vi "Host_SinglePointSuspension.vi"() -> ()   [LabVIEW 2024]
uses:
  <vilib>/FPGAPlugInAG/USB-7845R OEM/niLvFpga_Open_USB-7845R OEM.vi
  <vilib>/rvi/interface/common/dynamic/niFpgaDynamicAddResources.vi
  <vilib>/Utility/error.llb/Error Cluster From Error Code.vi
  <vilib>/rvi/errors/niLvFpgaAdjustHostInterfaceError.vi
  <vilib>/FPGAPlugInAG/Dynamic/niLvFpga_Close_Dynamic.vi
  <vilib>/rvi/interface/nirviOpenFPGA/nirviOpenFPGA.xnode
  FPGA Bitfiles/hoppingsicmv2_FPGATarget_FPGASinglePointS_HFntAzq5sS4.lvbitx
  <vilib>/rvi/interface/nirviReadWriteControl/nirviReadWriteControl.xnode
  <vilib>/rvi/interface/nirviCloseFPGA/nirviCloseFPGA.xnode
  NiFpgaLv.dll
  <vilib>/rvi/interface/Simulation/niFpgaSimulationCallBeginRW.vi
panel:
  in  "stop":bool
  in  "RetRate um/s":dbl format="%#_13g"
  in  "AppRate um/s":dbl format="%#_13g"
  in  "Retract um":dbl format="%#_13g"
  in  "Threshold %":dbl format="%#_13g"
  in  "Y um":dbl format="%#_13g"
  in  "X um":dbl format="%#_13g"
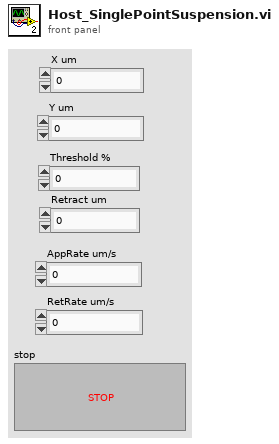
[diagram p1: front panel]
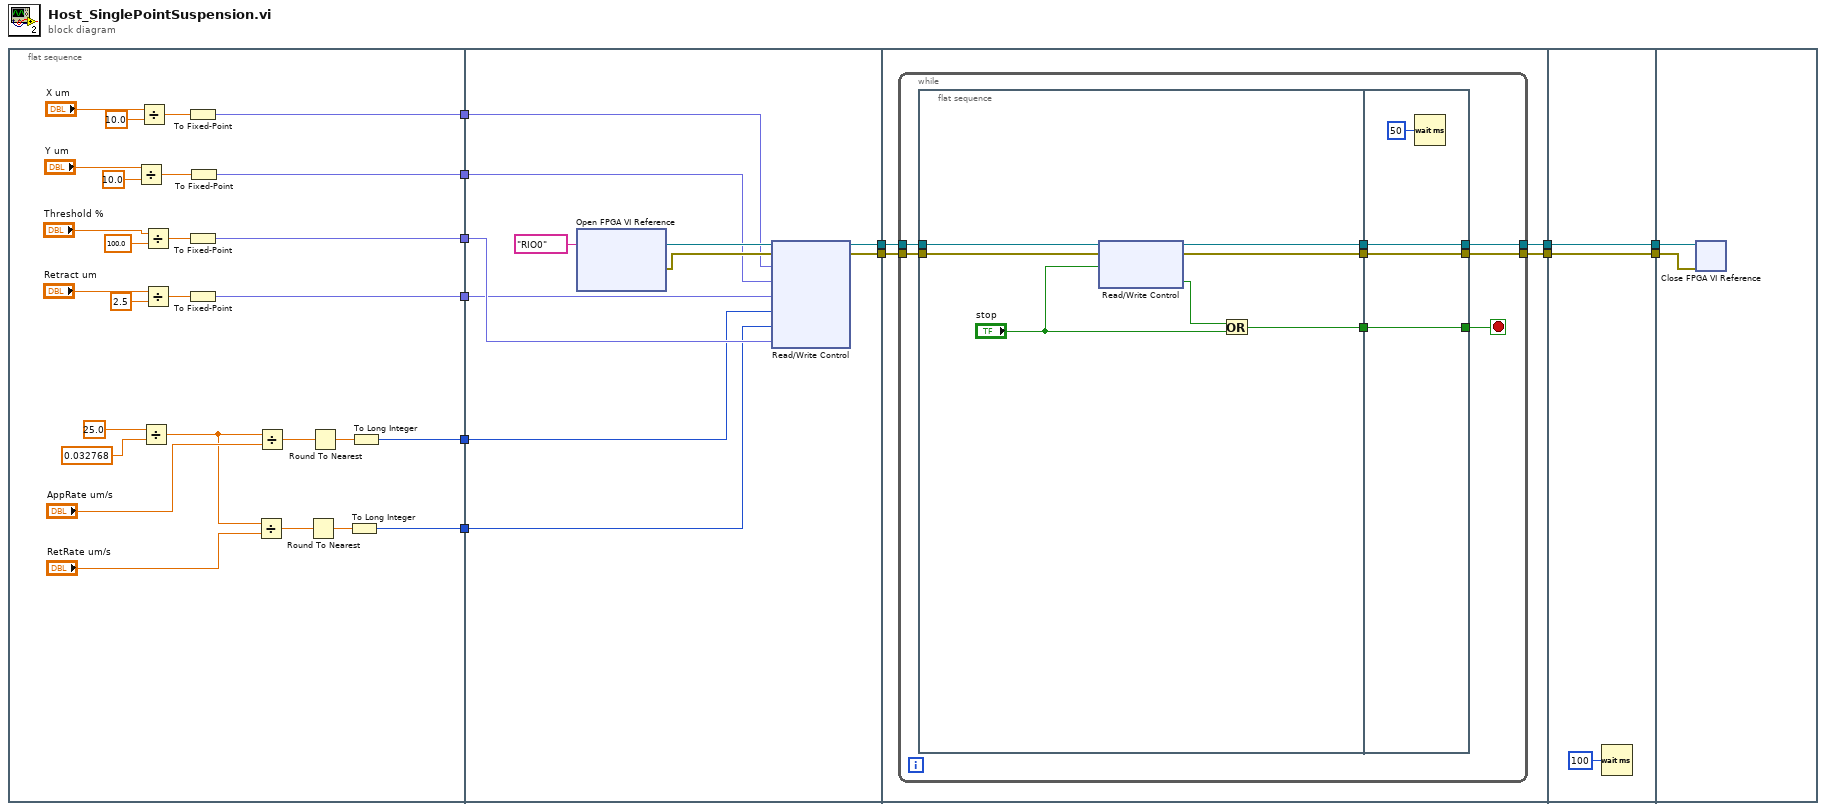
[diagram p0: block diagram]
diagram:
  n1 = flat-sequence {
    tunnel: [w36] -> w12
    tunnel: [w29] -> w11
    tunnel: [w28] -> w10
    tunnel: [w24] -> w9
    tunnel: [w14] -> w8
    tunnel: [w13] -> w7
    tunnel: w12 -> [w47]
    tunnel: w11 -> [w46]
    tunnel: w10 -> [w45]
    tunnel: w9 -> [w44]
    tunnel: w8 -> [w43]
    tunnel: w7 -> [w42]
    tunnel: [w41] -> w6
    tunnel: [w40] -> w5
    tunnel: w6 -> [w54]
    tunnel: w5 -> [w53]
    tunnel: [w52] -> w4
    tunnel: [w51] -> w3
    tunnel: w4 -> [w75]
    tunnel: w3 -> [w74]
    tunnel: [w75] -> w2
    tunnel: [w74] -> w1
    tunnel: w2 -> [w78]
    tunnel: w1 -> [w77]
    frame #0 {
      n2 = Divide(x="Y um", y=10.0) -> (x/y=w31:dbl)
      n3 = Divide(x="X um", y=10.0) -> (x/y=w30:dbl)
      n4 = Divide(x=25.0, y=0.032768) -> (x/y=w20:dbl)
      n5 = Divide(x="Threshold %", y=100.0) -> (x/y=w37:dbl)
      n6 = Divide(x="Retract um", y=2.5) -> (x/y=w27:dbl)
      n7 = To Fixed-Point(number=w30) -> (fixed-point=w29:fxp<+/-,48,16>)  [unwired: 1 in]
      n8 = To Fixed-Point(number=w37) -> (fixed-point=w36:fxp<+/-,48,16>)  [unwired: 1 in]
      n9 = To Fixed-Point(number=w27) -> (fixed-point=w24:fxp<+/-,48,16>)  [unwired: 1 in]
      n10 = To Fixed-Point(number=w31) -> (fixed-point=w28:fxp<+/-,48,16>)  [unwired: 1 in]
      n11 = Divide(x=w20, y="RetRate um/s") -> (x/y=w15:dbl)
      n12 = Divide(x=w20, y="AppRate um/s") -> (x/y=w17:dbl)
      n13 = Round To Nearest(number=w15) -> (nearest integer value=w16:dbl)
      n14 = Round To Nearest(number=w17) -> (nearest integer value=w18:dbl)
      n15 = To Long Integer(number=w16) -> (32bit integer=w13:i32)
      n16 = To Long Integer(number=w18) -> (32bit integer=w14:i32)
    }
    frame #1 {
      n17 = xnode "Open FPGA VI Reference"("resource name"=tag "RIO0") -> ("FPGA VI Reference Out"=w49:refnum<k20>, "error out"=w48:errorcluster)  [unwired: 1 in]
      n18 = xnode "Read/Write Control"("FPGA VI Reference In"=w49, "error in"=w48, "X"=w46, "Y"=w45, "Retract"=w44, "AppRate us"=w43, "RetRate us"=w42, "Threshold"=w47) -> ("FPGA VI Reference Out"=w41:refnum<k20>, "error out"=w40:errorcluster)
    }
    frame #2 {
      n19 = while {
        tunnel: w54 -> [w62]
        tunnel: w53 -> [w61]
        tunnel: [w58] -> w52
        tunnel: [w57] -> w51
        stop <- w55 stop-if-true
        n20 = flat-sequence {
          tunnel: w61 -> [w68]
          tunnel: w62 -> [w69]
          tunnel: [w67] -> w60
          tunnel: [w66] -> w59
          tunnel: [w63] -> w56
          tunnel: [w72] -> w58
          tunnel: w60 -> [w72]
          tunnel: w59 -> [w71]
          tunnel: [w71] -> w57
          tunnel: w56 -> [w70]
          tunnel: [w70] -> w55
          frame #0 {
            n21 = xnode "Read/Write Control"("FPGA VI Reference In"=w69, "error in"=w68, "stop"="stop") -> ("FPGA VI Reference Out"=w67:refnum<k20>, "error out"=w66:errorcluster, "TargetDone?"=w65:bool)
            n22 = Or(x=w65, y="stop") -> (x .or. y?=w63:bool)
          }
          frame #1 {
            n23 = Wait (ms)(milliseconds to wait=u32 50) -> ()  [unwired: 1 out]
          }
        }
      }
    }
    frame #3 {
      n24 = Wait (ms)(milliseconds to wait=u32 100) -> ()  [unwired: 1 out]
    }
    frame #4 {
      n25 = xnode "Close FPGA VI Reference"("FPGA VI Reference In"=w78, "error in"=w77) -> ()  [unwired: 1 out]
    }
  }
